vi "hse-application_GetApplicationInfos.vi"(8 "error in":errorcluster) -> (0 "error out":errorcluster, 1 "Application Name":string, 2 "Application Unit-ID":string, 3 "Application Title":string)   [LabVIEW 2014, in "hse-application.lvclass"]
doc: "Returns information on the application itself for display, logging, ...\n\n\n\n____\nHAMPEL SOFTWARE ENGINEERING v0.12.0 (2018-09-13 18:21)"
uses:
  hse-application.lvclass
  hse-application.lvclass/hse-application.ctl
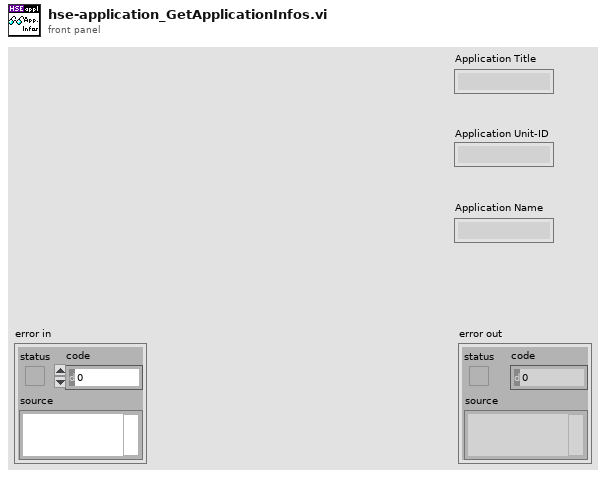
[diagram p1: front panel]
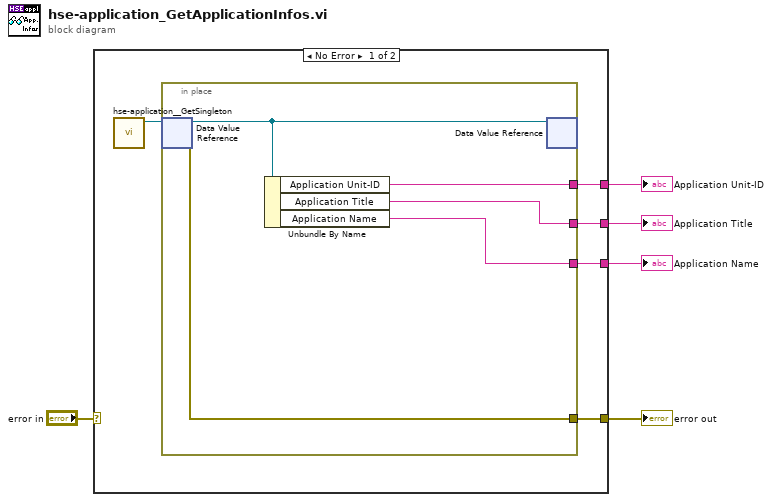
[diagram p0: block diagram]
diagram:
  n1 = case shown="No Error" "error in" {
    selector: "error in" -> [_ w16]
    tunnel: [w9 w16] -> w4
    tunnel: [w8 _] -> w3
    tunnel: [w7 _] -> w2
    tunnel: [w6 _] -> w1
    frame No Error {
      n2 = call "hse-application__GetSingleton.vi"() -> ("ApplicationClass DVR"=w10:refnum<data-value>)  [unwired: 10 in, 1 out]
      n3 = in-place {
        in-place-border: [w14] -> w9
        in-place-border: [w13] -> w8
        in-place-border: [w12] -> w7
        in-place-border: [w11] -> w6
        n4 = in-place-dvr #1(w10) -> (w15:refnum<class "hse-application.lvclass">, w14:errorcluster)
        n5 = Unbundle By Name(w15) -> ("Application Unit-ID"=w12:string, "Application Title"=w13:string, "Application Name"=w11:string)
        n6 = in-place-dvr #1(w15) -> ()  [unwired: 2 out]
      }
    }
    frame Error {
    }
  }
  "error out" <- w4
  "Application Title" <- w3
  "Application Unit-ID" <- w2
  "Application Name" <- w1
